vi "Verileri GUI'ye Gönder_UIM.vi"(1 "Sequence Context":refnum<k7>, 3 "Uygulanan Deðer":dbl, 4 "FD2 C":dbl, 5 "FD2 B":dbl, 6 "FD2 A":dbl, 7 "FD1 C":dbl, 8 "FD1 B":dbl, 9 "FD1 A":dbl, 10 "Limit Deger":dbl, 11 "Ölçüm No":u16) -> (0 "error out":errorcluster)   [LabVIEW 2014]
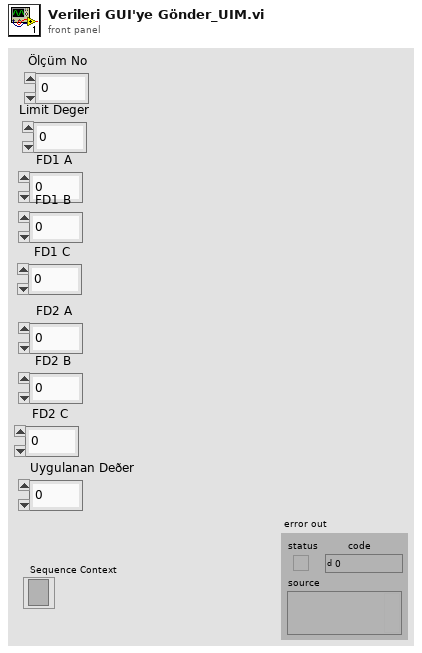
[diagram p1: front panel]
types:
  T1 = typedef "TestStand - Status Monitor.ctl" = cluster{"Sequence Context":refnum<k7>, "Execution":refnum<k7>, "Termination Monitor":refnum<k7>}
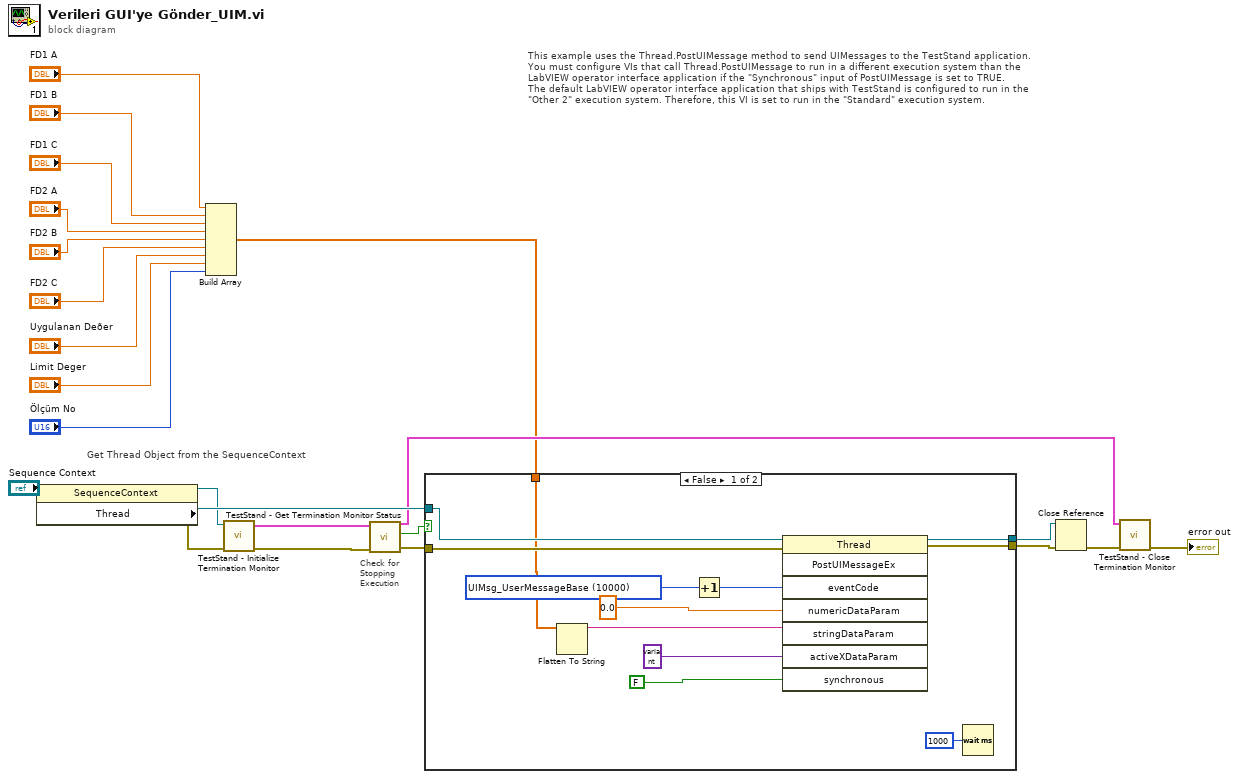
[diagram p0: block diagram]
diagram:
  # "Check for\nStopping\nExecution"
  # "This example uses the Thread.PostUIMessage method to send UIMessages to the TestStand application.  \nYou must configure VIs that call Thread.PostUIMessage to run in a different execution system than the\nLabVIEW operator interface application if the \"Synchronous\" input of PostUIMessage is set to TRUE.\nThe default LabVIEW operator interface application that ships with TestStand is configured to run in the\n\"Other 2\" execution system. Therefore, this VI is set to run in the \"Standard\" execution system."
  # "Get Thread Object from the SequenceContext"
  n1 = property class="SequenceContext"(reference="Sequence Context") -> (reference out=w19:refnum<k7>, error out=w18:errorcluster, "Thread"=w22:refnum<k7>)  [unwired: 1 in]
  n2 = Build Array("FD1 A", "FD1 B", "FD1 C", "FD2 A", "FD2 B", "FD2 C", "Uygulanan Deðer", "Limit Deger", "Ölçüm No") -> (w1:dbl[])
  n3 = call <vilib>:"TestStand - Initialize Termination Monitor.vi"("error in (no error)"=w18, "Sequence Context In"=w19) -> ("error out"=w17:errorcluster, "Status Monitor Out"=w16:T1)  [unwired: 8 out]
  n4 = call <vilib>:"TestStand - Get Termination Monitor Status.vi"("error in (no error)"=w17, "Status Monitor In"=w16) -> ("error out"=w12:errorcluster, "Terminating or Aborting"=w11:bool, "Status Monitor Out"=w14:T1)  [unwired: 7 out]
  n5 = case shown="False" w11 {
    tunnel: w22 -> [w35 w36]
    tunnel: [w31 w36] -> w20
    tunnel: [w30 w37] -> w21
    tunnel: w12 -> [w33 w37]
    tunnel: w1 -> [w28 _]
    frame False {
      w25 = 10000 items=["UIMsg_BreakOnUserRequest"=1, "UIMsg_BreakOnBreakpoint"=2, "UIMsg_BreakOnRunTimeError"=3, "UIMsg_Trace"=4, "UIMsg_TerminatingExecution"=5, "UIMsg_AbortingExecution"=6, "UIMsg_KillingExecutionThreads"=7, "UIMsg_EndExecution"=8, "UIMsg_ShutDownComplete"=9, "UIMsg_StartExecution"=10, "UIMsg_ProgressPercent"=11, "UIMsg_ProgressText"=12, "UIMsg_StartInteractiveExecution"=13, "UIMsg_EndInteractiveExecution"=14, "UIMsg_TerminatingInteractiveExecution"=15, "UIMsg_TerminationCancelled"=16, "UIMsg_ResumeFromBreak"=17, "UIMsg_StartFileExecution"=18, "UIMsg_EndFileExecution"=19, "UIMsg_ShutDownCancelled"=20, "UIMsg_LocalizationSettingChanged"=21, "UIMsg_OpenWindows"=22, "UIMsg_TileWindows"=23, "UIMsg_CascadeWindows"=24, "UIMsg_ReportChanged"=25, "UIMsg_CloseWindows"=26, "UIMsg_RefreshWindows"=27, "UIMsg_ClientFileChanged"=28, "UIMsg_DisplayReport"=29, "UIMsg_ModelState_Initializing"=30, "UIMsg_ModelState_Waiting"=31, "UIMsg_ModelState_Identified"=32, "UIMsg_ModelState_BeginTesting"=33, "UIMsg_ModelState_TestingComplete"=34, "UIMsg_ModelState_PostProcessingComplete"=35, "UIMsg_ModelState_EnabledStateSet"=36, "UIMsg_ReportLocationChanged"=37, "UIMsg_GotoLocation"=38, "UIMsg_PushUndoItem"=39, "UIMsg_OutputMessages"=40, "UIMsg_TypePaletteFileListChanged"=41, "UIMsg_NonTerminatableThreadsArePreventingTermination"=42, "UIMsg_ModelState_PostProcessing"=43, "UIMsg_ReportCollectionChanged"=44, "UIMsg_RuntimeError"=45, "UIMsg_UserMessageBase"=10000] ("eventCode")
      n6 = Flatten To String(anything=w28) -> (data string=w27:string)  [unwired: 3 in, 2 out]
      n7 = Increment(x=w25) -> (x+1=w24:i32)
      n8 = invoke class="Thread" method="PostUIMessageEx"(reference=w35, error in=w33, "eventCode"=w24, "numericDataParam"=0.0, "stringDataParam"=w27, "activeXDataParam"=variant, "synchronous"=FALSE) -> (reference out=w31:refnum<k7>, error out=w30:errorcluster)  [unwired: 1 in, 6 out]
      n9 = Wait (ms)(milliseconds to wait=u32 1000) -> ()  [unwired: 1 out]
    }
    frame True {
    }
  }
  n10 = Close Reference(reference=w20, error in (no error)=w21) -> (error out=w15:errorcluster)
  n11 = call <vilib>:"TestStand - Close Termination Monitor.vi"("error in (no error)"=w15, "Status Monitor In"=w14) -> ("error out"=→"error out":errorcluster)  [unwired: 9 out]
